vi "QuickTest.vi"() -> ()   [LabVIEW 2016]
uses:
  Remote System/Remote System.lvclass
  C:/Program Files (x86)/National Instruments/LabVIEW 2016/vi.lib/LIEF/Forms/Shape/Shape.lvclass
  <vilib>/LIEF/Forms/Shape/Shape.lvclass
  <vilib>/LIEF/Image Editor Handler/Image Editor Handler.lvclass
panel:
  in  "2D Picture":picture
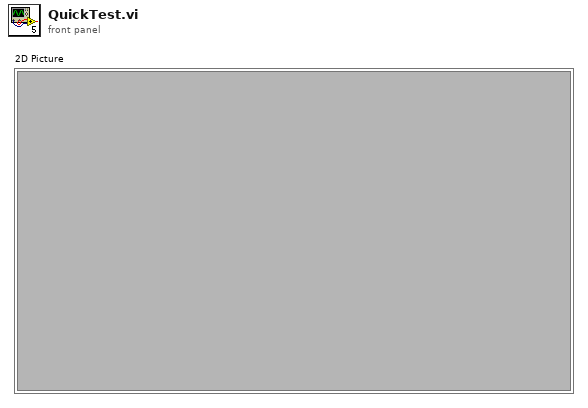
[diagram p1: front panel]
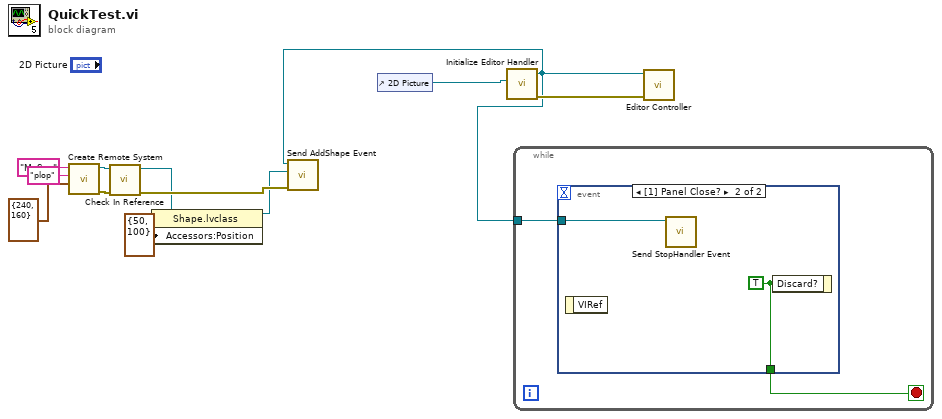
[diagram p0: block diagram]
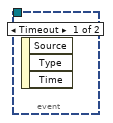
[diagram p2: hidden frame]
diagram:
  n1 = call "Create Remote System.vi"("Size"=cluster{"Width":i32, "Height":i32} {"Width"=240, "Height"=160}, "IP Address"="plop", "System Alias"="MySys") -> ("error out"=w9:errorcluster, "Remote System out"=w8:refnum<class "Remote System.lvclass">)  [unwired: 7 in]
  n2 = call <vilib>:"Check In Reference.vi"("error in (no error)"=w9, "Shape in"=w8) -> ("error out"=w7:errorcluster, "Shape Reference"=w6:refnum<data-value>)  [unwired: 8 in]
  n3 = property class="Shape.lvclass"(reference=w6, "Accessors:Position"=cluster{"Left":i32, "Top":i32} {"Left"=50, "Top"=100} ("Position")) -> (reference out=w5:refnum<data-value>)  [unwired: 1 in, 1 out]
  n4 = control-ref of="2D Picture"() -> (w12:refnum<vi>)
  n5 = call <vilib>:"Initialize Editor Handler.vi"("PictureRef"=w12) -> ("error out"=w11:errorcluster, "Editor Handler out"=w10:refnum<class "Image Editor Handler.lvclass">)  [unwired: 9 in]
  n6 = call <vilib>:"Send AddShape Event.vi"("error in (no error)"=w7, "New Shape Reference"=w5, "Editor Handler in"=w10) -> ()  [unwired: 7 in, 2 out]
  n7 = while {
    tunnel: w10 -> [w13]
    stop <- w14 stop-if-true
    n8 = event shown="[1] Panel Close?" {
      selector: _ -> [_ _]
      dyn-events: _ -> [_ _]
      timeout: _ -> [_ _]
      tunnel: [_ w16] -> w14
      tunnel: w13 -> [_ w15]
      event Timeout {
        n9 = event-data() -> ()  [unwired: 1 in, 3 out]
      }
      event Panel Close? {
        w16 = TRUE ("Discard?")
        n10 = event-data() -> ()  [unwired: 1 in, 1 out]
        n11 = call <vilib>:"Send StopHandler Event.vi"("Editor Handler in"=w15) -> ()  [unwired: 9 in, 2 out]
        n12 = event-data("Discard?"=w16) -> ()  [unwired: 1 in, 1 out]
      }
    }
  }
  n13 = call <vilib>:"Editor Controller.vi"("error in (no error)"=w11, "Editor Handler in"=w10) -> ()  [unwired: 8 in, 2 out]
